vi "Launch Nested Error Reporter Actor.vi"(8 "error in (no error)":errorcluster, 10 "Nested Actor in":refnum<class "Error Reporter.lvclass">, 11 "Caller Actor in":refnum<class "Error Reporter.lvclass">) -> (0 "error out":errorcluster, 2 "Nested Actor's Enqueuer":refnum<class "Message Enqueuer.lvclass">, 3 "Caller Actor out":refnum<class "Error Reporter.lvclass">)   [LabVIEW 2024, in "Error Reporter.lvlib" / "Error Reporter.lvclass"]
uses:
  Error Reporter.lvclass
  Error Reporter.lvclass/Error Reporter.ctl
  <vilib>/ActorFramework/Actor/Actor.lvclass
  <vilib>/ActorFramework/Message Enqueuer/Message Enqueuer.lvclass
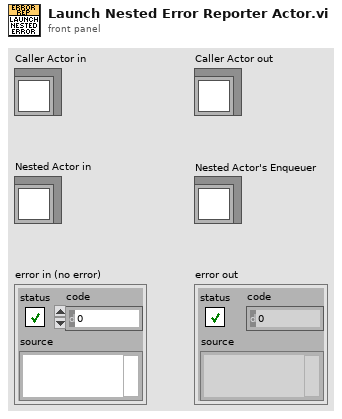
[diagram p1: front panel]
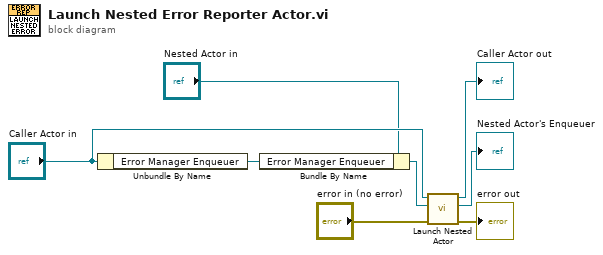
[diagram p0: block diagram]
diagram:
  n1 = Unbundle By Name("Caller Actor in") -> ("Error Manager Enqueuer"=w2:refnum<class "Message Enqueuer.lvclass">)
  n2 = Bundle By Name(cluster="Nested Actor in", "Error Manager Enqueuer"=w2) -> (w1:refnum<class "Error Reporter.lvclass">)
  n3 = call <vilib>:"Launch Nested Actor.vi"("error in (no error)"="error in (no error)", "Nested Actor"=w1, "Caller Actor in"="Caller Actor in") -> ("error out"=→"error out":errorcluster, "Nested Actor's Enqueuer"=→"Nested Actor's Enqueuer":refnum<class "Message Enqueuer.lvclass">, "Caller Actor out"=→"Caller Actor out":refnum<class "Error Reporter.lvclass">)  [unwired: 6 in]
